vi "DequeueManualMode.vi"(8 "error in (no error)":errorcluster, 10 "Acquire":bool, 11 "Queue in":refnum<queue>) -> (0 "error out":errorcluster, 2 "Data":variant, 3 "PreCollectionMessage":T1)   [LabVIEW 2019, in "ManualMode.lvlib"]
uses:
  ManualMode.lvlib
  Enum - ManualModeMessage.ctl
  Cluster - ManualModeMessageCluster.ctl
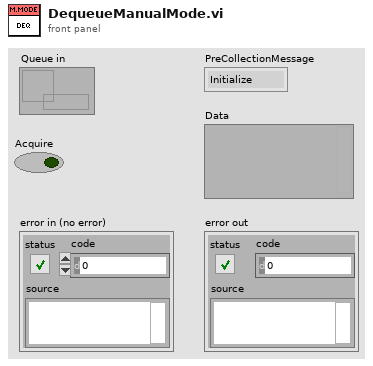
[diagram p1: front panel]
types:
  T1 = typedef "ManualMode.lvlib/Enum - ManualModeMessage.ctl" = enum16{"Initialize", "Idle", "Start", "Stop", "BroadcastPreCollection", "MoveCCW", "MoveCW", "StopMove", "SetZero", "GotoZero", "UpdateHW", "Error", "Exit"}
  T2 = typedef "ManualMode.lvlib/Cluster - ManualModeMessageCluster.ctl" = cluster{"Message":T1, "Data":variant}
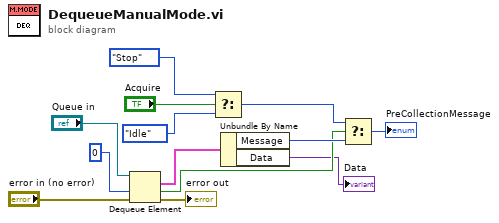
[diagram p0: block diagram]
diagram:
  n1 = Dequeue Element(queue="Queue in", timeout in ms (-1)=0, error in (no error)="error in (no error)") -> (element=w4:T2, timed out?=w10:bool, error out=→"error out":errorcluster)  [unwired: 1 out]
  n2 = Select(t=Enum_-_ManualModeMessage."Stop" ("y"), s="Acquire", f=Enum_-_ManualModeMessage."Idle" ("PreCollectionMessage")) -> (s? t:f=w11:T1)
  n3 = Unbundle By Name(w4) -> ("Message"=w12:T1, "Data"=→"Data":variant)
  n4 = Select(t=w11, s=w10, f=w12) -> (s? t:f=→"PreCollectionMessage":T1)
